vi "Get Controllers via Storage API.vi"(6 "Action":enum16{"PID", "Industrial"}(ring), 7 "VI reference (current VI)":refnum<vi>, 8 "error in (no error)":errorcluster, 10 "Tree":refnum<vi>, 11 "NIVS.System Definition Root":refnum<k24>) -> (0 "error out":errorcluster, 3 "NIVS.System Definition Root":refnum<k24>)   [LabVIEW 2019, in "Control Workspace Object.lvlib"]
uses:
  NationalInstruments.VeriStand.SystemStorage
  <vilib>/picture/picture.llb/imagedata.ctl
  Shared/Constants.vi
  Control Workspace Object.lvlib
  Workspace Shared/Control Workspace Shared.lvlib
  NationalInstruments.VeriStand.SystemDefinitionAPI
  Shared/Control Addon Shared.lvlib
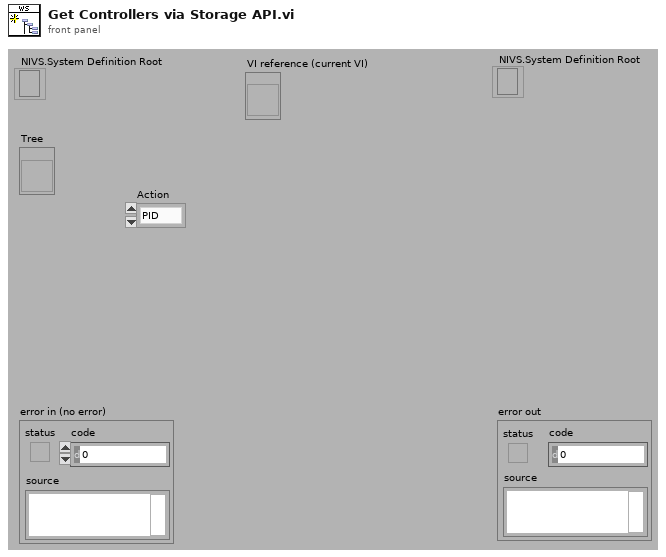
[diagram p1: front panel]
types:
  T1 = typedef "imagedata.ctl" = cluster{"image type":i32, "image depth":i32, "image":u8[], "mask":u8[], "colors":u32[], "Rectangle":cluster{"left":i16, "top":i16, "right":i16, "bottom":i16}}
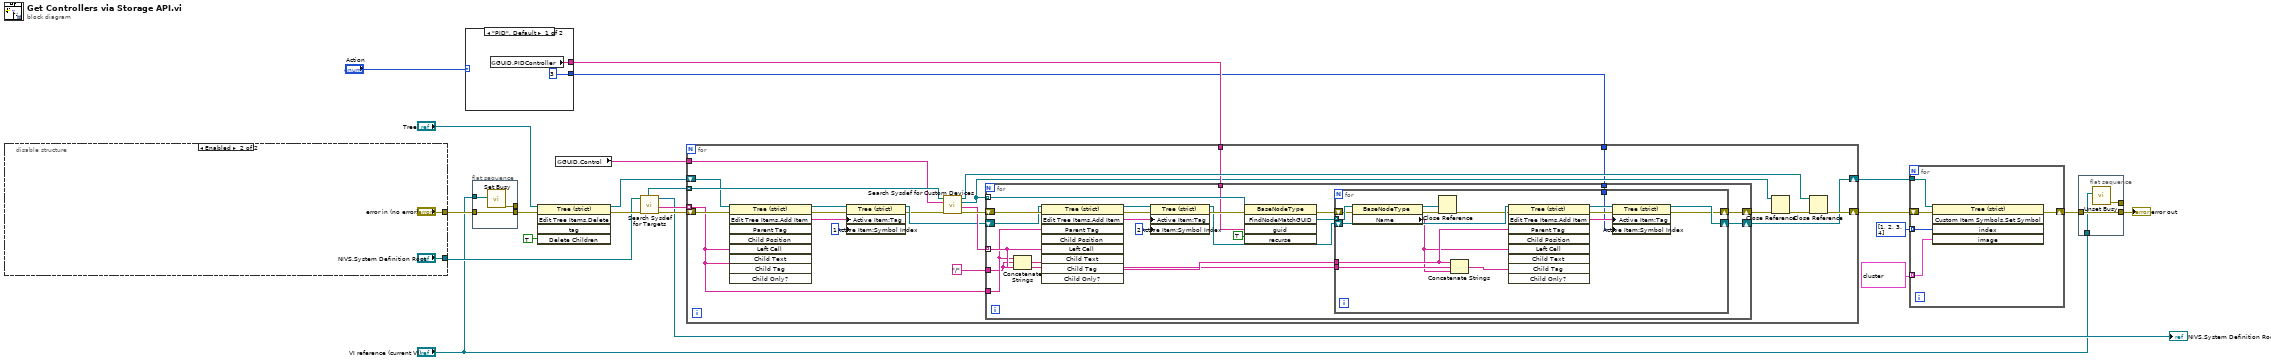
[diagram p0: block diagram]
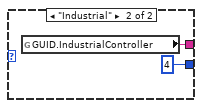
[diagram p2: hidden frame]
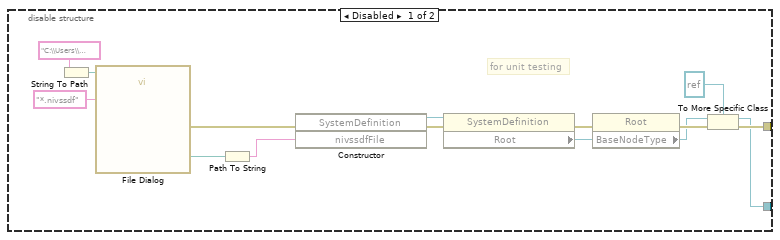
[diagram p3: hidden frame]
diagram:
  n1 = disable-structure shown="Enabled" {
    disable-tunnel: [w24 "NIVS.System Definition Root"] -> w14
    disable-tunnel: [w29 "error in (no error)"] -> w6
    frame Disabled {
      # "for unit testing"
      n2 = String To Path(string="C:\\Users\\Public\\Documents\\National Instruments\\NI VeriStand 2010\\Projects") -> (path=w25:path)
      n3 = call "File Dialog"("start path"=w25, "pattern (all files)"="*.nivssdf") -> ("selected path"=w36:path, "error out"=w23:errorcluster)  [unwired: 10 in, 2 out]
      n4 = Path To String(path=w36) -> (string=w35:string)
      n5 = constructor class="SystemDefinition"(error in=w23, "nivssdfFile"=w35) -> (reference out=w33:refnum<k24>, error out=w34:errorcluster)  [unwired: 2 in, 2 out]
      n6 = property class="SystemDefinition"(reference=w33, error in=w34) -> (error out=w31:errorcluster, "Root"=w32:refnum<k24>)  [unwired: 1 out]
      n7 = property class="Root"(reference=w32, error in=w31) -> (error out=w30:errorcluster, "BaseNodeType"=w28:refnum<k24>)  [unwired: 1 out]
      n8 = To More Specific Class(target class=refnum<k24> refnum, reference=w28, error in=w30) -> (specific class reference=w24:refnum<k24>, error out=w29:errorcluster)
    }
    frame Enabled {
    }
  }
  n9 = case shown="\"PID\", Default" "Action" {
    tunnel: [w41 w43] -> w4
    tunnel: [3 4] -> w2
    frame "PID", Default {
      n10 = global read "Constants.vi" "GUID.PIDController"() -> (w41:string)
    }
    frame "Industrial" {
      n11 = global read "Constants.vi" "GUID.IndustrialController"() -> (w43:string)
    }
  }
  n12 = flat-sequence {
    tunnel: [w45] -> w20
    tunnel: "VI reference (current VI)" -> [w46]
    tunnel: w6 -> [w45]
    tunnel: [w44] -> _
    frame #0 {
      n13 = call <vilib>:"Set Busy.vi"("VI reference (current VI)"=w46) -> ("error out"=w44:errorcluster)  [unwired: 9 in, 1 out]
    }
  }
  n14 = invoke class="Tree (strict)" method="Edit Tree Items.Delete"(reference="Tree", error in=w20, "Delete Children"=TRUE ("Delete Children?")) -> (reference out=w13:refnum<vi>, error out=w19:errorcluster)  [unwired: 2 in, 3 out]
  n15 = global read "Constants.vi" "GUID.Control"() -> (w1:string)
  n16 = call "Search Sysdef for Targets.vi"("error in (no error)"=w19, "NIVS.System Definition Root"=w14) -> ("error out"=w18:errorcluster, "Target Names"=w22:string[], "NIVS.System Defintion Root Out"=→"NIVS.System Definition Root":refnum<k24>, "Target Nodes"=w17:refnum<k24>[])  [unwired: 6 in]
  n17 = for {
    tunnel: w17 -> [w67] mode=indexing
    tunnel: w22 -> [w60] mode=indexing
    shift-right: [w62] -> w11
    shift-left: w18 -> [w68]
    tunnel: w1 -> [w58]
    shift-right: [w51] -> w12
    shift-left: w13 -> [w50]
    tunnel: w4 -> [w49]
    tunnel: w2 -> [w47]
    n18 = invoke class="Tree (strict)" method="Edit Tree Items.Add Item"(reference=w50, error in=w68, "Left Cell"=w60, "Child Tag"=w60) -> (reference out=w56:refnum<vi>, error out=w53:errorcluster, "Edit Tree Items:Add Item"=w54:string)  [unwired: 5 in, 6 out]
    n19 = property class="Tree (strict)"(reference=w56, error in=w53, "Active Item:Tag"=w54, "Active Item:Symbol Index"=1) -> (reference out=w55:refnum<vi>, error out=w52:errorcluster)
    n20 = call "Search Sysdef for Custom Devices.vi"("error in (no error)"=w52, "CD GUID"=w58, "Target Node"=w67) -> ("error out"=w66:errorcluster, "Custom Device Names"=w65:string[], "Custom Device Nodes"=w48:refnum<k24>[], "Target Node Out"=w61:refnum<k24>)  [unwired: 5 in]
    n21 = for {
      tunnel: w65 -> [w87] mode=indexing
      tunnel: w60 -> [w85]
      shift-right: [w73] -> w64
      shift-left: w66 -> [w88]
      tunnel: "/" ("string") -> [w70]
      shift-right: [w75] -> w51
      shift-left: w55 -> [w86]
      tunnel: w48 -> [w80] mode=indexing
      tunnel: w49 -> [w77]
      tunnel: w47 -> [w69]
      n22 = Concatenate Strings(w85, w70, w87) -> (w71:string)
      n23 = invoke class="Tree (strict)" method="Edit Tree Items.Add Item"(reference=w86, error in=w88, "Parent Tag"=w85, "Left Cell"=w87, "Child Tag"=w71) -> (reference out=w83:refnum<vi>, error out=w81:errorcluster, "Edit Tree Items:Add Item"=w82:string)  [unwired: 4 in, 6 out]
      n24 = property class="Tree (strict)"(reference=w83, error in=w81, "Active Item:Tag"=w82, "Active Item:Symbol Index"=2) -> (reference out=w76:refnum<vi>, error out=w79:errorcluster)
      n25 = invoke class="BaseNodeType" method="FindNodeMatchGUID"(reference=w80, error in=w79, "guid"=w77, "recurse"=TRUE) -> (error out=w74:errorcluster, "FindNodeMatchGUID"=w72:refnum<k24>[])  [unwired: 1 in, 3 out]
      n26 = for {
        shift-right: [w93] -> w75
        shift-left: w76 -> [w104]
        shift-right: [w91] -> w73
        shift-left: w74 -> [w102]
        tunnel: w72 -> [w103] mode=indexing
        tunnel: w71 -> [w100]
        tunnel: w70 -> [w99]
        tunnel: w69 -> [w89]
        n27 = property class="BaseNodeType"(reference=w103, error in=w102) -> (reference out=w95:refnum<k24>, error out=w101:errorcluster, "Name"=w98:string)
        n28 = Close Reference(reference=w95, error in (no error)=w101) -> (error out=w96:errorcluster)
        n29 = Concatenate Strings(w100, w99, w98) -> (w97:string)
        n30 = invoke class="Tree (strict)" method="Edit Tree Items.Add Item"(reference=w104, error in=w96, "Parent Tag"=w100, "Left Cell"=w98, "Child Tag"=w97) -> (reference out=w94:refnum<vi>, error out=w92:errorcluster, "Edit Tree Items:Add Item"=w90:string)  [unwired: 4 in, 6 out]
        n31 = property class="Tree (strict)"(reference=w94, error in=w92, "Active Item:Tag"=w90, "Active Item:Symbol Index"=w89) -> (reference out=w93:refnum<vi>, error out=w91:errorcluster)
      }
    }
    n32 = Close Reference(reference=w48, error in (no error)=w64) -> (error out=w63:errorcluster)
    n33 = Close Reference(reference=w61, error in (no error)=w63) -> (error out=w62:errorcluster)
  }
  n34 = for {
    tunnel: w12 -> [w109]
    shift-right: [w108] -> w9
    shift-left: w11 -> [w106]
    tunnel: i32[] [1, 2, 3, 4] -> [w107] mode=indexing
    tunnel: T1[] [{"image type"=0, "image depth"=32, "image"=array[1024 elements], "mask"=[0, 0, 0, 0, 0, 0, 63, 254, 127, 254, 255, 254, 255, 255, 255, 255, 255, 255, 255, 255, 255, 255, 255, 255, 127, 254, 64, 32, 0, 0, 0, 0], "colors"=[], "Rectangle"={"left"=0, "top"=0, "right"=16, "bottom"=16}}, {"image type"=0, "image depth"=32, "image"=array[1024 elements], "mask"=[255, 255, 255, 255, 255, 255, 255, 255, 255, 255, 255, 255, 255, 255, 255, 255, 255, 255, 255, 255, 255, 255, 255, 255, 255, 255, 255, 255, 255, 255, 255, 255], "colors"=[], "Rectangle"={"left"=0, "top"=0, "right"=16, "bottom"=16}}, {"image type"=0, "image depth"=32, "image"=[255, 255, 255, 255, 255, 255, 255, 255, 255, 255, 255, 255, 255, 255, 255, 255, 255, 255, 255, 255, 255, 255, 255, 255, 255, 0, 0, 0, 255, 0, 0, 0, 255, 0, 0, 0, 255, 0, 0, 0, 255, 255, 255, 255, 255, 255, 255, 255, 255, 255, 255, 255, 255, 255, 255, 255, 255, 255, 255, 255, 255, 255, 255, 255, 255, 255, 255, 255, 255, 255, 255, 255, 255, 247, 247, 247, 255, 255, 255, 255, 255, 0, 0, 0, 255, 0, 0, 0, 255, 0, 0, 0, 255, 0, 0, 0, 255, 0, 0, 0, 255, 0, 0, 0, 255, 0, 0, 0, 255, 0, 0, 0, 255, 255, 255, 255, 255, 248, 248, 248, 255, 255, 255, 255, 255, 255, 255, 255, 255, 255, 255, 255, 255, 255, 255, 255, 255, 255, 255, 255, 255, 0, 0, 0, 255, 0, 0, 0, 255, 0, 0, 0, 255, 0, 0, 0, 255, 0, 0, 0, 255, 0, 0, 0, 255, 0, 0, 0, 255, 0, 0, 0, 255, 0, 0, 0, 255, 0, 0, 0, 255, 255, 255, 255, 255, 249, 249, 249, 255, 254, 254, 254, 255, 255, 255, 255, 255, 255, 255, 255, 255, 0, 0, 0, 255, 0, 0, 0, 255, 0, 0, 0, 255, 0, 0, 0, 255, 0, 0, 0, 255, 0, 0, 0, 255, 0, 0, 0, 255, 0, 0, 0, 255, 0, 0, 0, 255, 0, 0, 0, 255, 0, 0, 0, 255, 0, 0, 0, 255, 255, 255, 255, 255, 255, 255, 255, 255, 255, 255, 255, 255, 0, 0, 0, 255, 0, 0, 0, 255, 0, 0, 0, 255, 0, 0, 0, 255, 0, 0, 0, 255, 0, 0, 0, 255, 0, 0, 0, 255, 0, 0, 0, 255, 0, 0, 0, 255, 0, 0, 0, 255, 0, 0, 0, 255, 0, 0, 0, 255, 0, 0, 0, 255, 0, 0, 0, 255, 255, 255, 255, 255, 255, 255, 255, 255, 0, 0, 0, 255, 0, 0, 0, 255, 255, 255, 255, 255, 255, 255, 255, 255, 255, 255, 255, 255, 255, 255, 255, 255, 255, 255, 255, 255, 255, 255, 255, 255, 255, 255, 255, 255, 255, 255, 255, 255, 255, 255, 255, 255, 255, 255, 255, 255, 0, 0, 0, 255, 0, 0, 0, 255, 255, 255, 255, 255, 0, 0, 0, 255, 0, 0, 0, 255, 0, 0, 0, 255, 255, 255, 255, 255, 0, 0, 0, 255, 0, 0, 0, 255, 0, 0, 0, 255, 0, 0, 0, 255, 0, 0, 0, 255, 0, 0, 0, 255, 0, 0, 0, 255, 0, 0, 0, 255, 242, 242, 242, 255, 0, 0, 0, 255, 0, 0, 0, 255, 0, 0, 0, 255, 0, 0, 0, 255, 0, 0, 0, 255, 0, 0, 0, 255, 255, 255, 255, 255, 0, 0, 0, 255, 0, 0, 0, 255, 0, 0, 0, 255, 0, 0, 0, 255, 0, 0, 0, 255, 0, 0, 0, 255, 0, 0, 0, 255, 0, 0, 0, 255, 255, 255, 255, 255, 0, 0, 0, 255, 0, 0, 0, 255, 0, 0, 0, 255, 0, 0, 0, 255, 0, 0, 0, 255, 0, 0, 0, 255, 255, 255, 255, 255, 0, 0, 0, 255, 0, 0, 0, 255, 0, 0, 0, 255, 0, 0, 0, 255, 0, 0, 0, 255, 0, 0, 0, 255, 255, 255, 255, 255, 0, 0, 0, 255, 255, 255, 255, 255, 0, 0, 0, 255, 0, 0, 0, 255, 0, 0, 0, 255, 0, 0, 0, 255, 0, 0, 0, 255, 0, 0, 0, 255, 255, 255, 255, 255, 0, 0, 0, 255, 0, 0, 0, 255, 0, 0, 0, 255, 0, 0, 0, 255, 0, 0, 0, 255, 255, 255, 255, 255, 255, 255, 255, 255, 0, 0, 0, 255, 255, 255, 255, 255, 0, 0, 0, 255, 0, 0, 0, 255, 0, 0, 0, 255, 255, 255, 255, 255, 0, 0, 0, 255, 0, 0, 0, 255, 255, 255, 255, 255, 255, 255, 255, 255, 255, 255, 255, 255, 0, 0, 0, 255, 0, 0, 0, 255, 255, 255, 255, 255, 255, 255, 255, 255, 255, 255, 255, 255, 255, 255, 255, 255, 255, 255, 255, 255, 0, 0, 0, 255, 0, 0, 0, 255, 255, 255, 255, 255, 255, 255, 255, 255, 0, 0, 0, 255, 0, 0, 0, 255, 0, 0, 0, 255, 0, 0, 0, 255, 0, 0, 0, 255, 0, 0, 0, 255, 0, 0, 0, 255, 0, 0, 0, 255, 255, 255, 255, 255, 255, 255, 255, 255, 0, 0, 0, 255, 0, 0, 0, 255, 0, 0, 0, 255, 0, 0, 0, 255, 255, 255, 255, 255, 255, 255, 255, 255, 255, 255, 255, 255, 0, 0, 0, 255, 0, 0, 0, 255, 0, 0, 0, 255, 0, 0, 0, 255, 0, 0, 0, 255, 0, 0, 0, 255, 0, 0, 0, 255, 0, 0, 0, 255, 255, 255, 255, 255, 0, 0, 0, 255, 0, 0, 0, 255, 0, 0, 0, 255, 255, 255, 255, 255, 254, 254, 254, 255, 255, 255, 255, 255, 255, 255, 255, 255, 255, 255, 255, 255, 0, 0, 0, 255, 0, 0, 0, 255, 0, 0, 0, 255, 0, 0, 0, 255, 0, 0, 0, 255, 0, 0, 0, 255, 0, 0, 0, 255, 0, 0, 0, 255, 0, 0, 0, 255, 0, 0, 0, 255, 255, 255, 255, 255, 255, 255, 255, 255, 255, 255, 255, 255, 255, 255, 255, 255, 255, 255, 255, 255, 249, 249, 249, 255, 255, 255, 255, 255, 0, 0, 0, 255, 0, 0, 0, 255, 0, 0, 0, 255, 0, 0, 0, 255, 0, 0, 0, 255, 0, 0, 0, 255, 0, 0, 0, 255, 0, 0, 0, 255, 255, 255, 255, 255, 255, 255, 255, 255, 248, 248, 248, 255, 251, 251, 251, 255, 255, 255, 255, 255, 255, 255, 255, 255, 255, 255, 255, 255, 252, 252, 252, 255, 255, 255, 255, 255, 255, 255, 255, 255, 0, 0, 0, 255, 0, 0, 0, 255, 0, 0, 0, 255, 0, 0, 0, 255, 255, 255, 255, 255, 255, 255, 255, 255, 254, 254, 254, 255, 252, 252, 252, 255, 251, 251, 251, 255, 252, 252, 252], "mask"=[255, 255, 255, 255, 255, 255, 255, 255, 255, 255, 255, 255, 255, 255, 255, 255, 255, 255, 255, 255, 255, 255, 255, 255, 255, 255, 255, 255, 255, 255, 255, 255], "colors"=[], "Rectangle"={"left"=0, "top"=0, "right"=16, "bottom"=16}}, {"image type"=0, "image depth"=32, "image"=[255, 255, 255, 255, 255, 255, 255, 255, 255, 255, 255, 255, 255, 255, 255, 255, 255, 255, 255, 255, 255, 255, 255, 255, 255, 0, 0, 0, 255, 0, 0, 0, 255, 0, 0, 0, 255, 0, 0, 0, 255, 255, 255, 255, 255, 255, 255, 255, 255, 255, 255, 255, 255, 255, 255, 255, 255, 255, 255, 255, 255, 255, 255, 255, 255, 255, 255, 255, 255, 255, 255, 255, 255, 255, 255, 255, 255, 255, 255, 255, 255, 0, 0, 0, 255, 0, 0, 0, 255, 0, 0, 0, 255, 8, 8, 8, 255, 0, 0, 0, 255, 1, 1, 1, 255, 0, 0, 0, 255, 1, 1, 1, 255, 255, 255, 255, 255, 247, 247, 247, 255, 255, 255, 255, 255, 255, 255, 255, 255, 255, 255, 255, 255, 255, 255, 255, 255, 255, 255, 255, 255, 0, 0, 0, 255, 0, 0, 0, 255, 0, 0, 0, 255, 9, 9, 9, 255, 255, 255, 255, 255, 255, 255, 255, 255, 0, 0, 0, 255, 0, 0, 0, 255, 0, 0, 0, 255, 0, 0, 0, 255, 255, 255, 255, 255, 248, 248, 248, 255, 254, 254, 254, 255, 255, 255, 255, 255, 255, 255, 255, 255, 0, 0, 0, 255, 0, 0, 0, 255, 0, 0, 0, 255, 255, 255, 255, 255, 11, 11, 10, 255, 255, 255, 255, 255, 255, 255, 255, 255, 7, 7, 7, 255, 255, 255, 255, 255, 0, 0, 0, 255, 0, 0, 0, 255, 0, 0, 0, 255, 255, 255, 255, 255, 255, 255, 255, 255, 255, 255, 255, 255, 0, 0, 0, 255, 0, 0, 0, 255, 0, 0, 0, 255, 255, 255, 255, 255, 255, 255, 255, 255, 7, 7, 7, 255, 255, 255, 255, 255, 255, 255, 255, 255, 0, 0, 0, 255, 255, 255, 255, 255, 254, 254, 254, 255, 0, 0, 0, 255, 4, 4, 3, 255, 0, 0, 0, 255, 255, 255, 255, 255, 255, 255, 255, 255, 0, 0, 0, 255, 0, 0, 0, 255, 243, 243, 243, 255, 255, 255, 255, 255, 0, 0, 0, 255, 7, 7, 7, 255, 255, 255, 255, 255, 255, 255, 255, 255, 0, 0, 0, 255, 0, 0, 0, 255, 255, 255, 255, 255, 255, 255, 255, 255, 0, 0, 0, 255, 0, 0, 0, 255, 255, 255, 255, 255, 0, 0, 0, 255, 0, 0, 0, 255, 0, 0, 0, 255, 255, 255, 255, 255, 0, 0, 0, 255, 0, 0, 0, 255, 0, 0, 0, 255, 0, 0, 0, 255, 0, 0, 0, 255, 0, 0, 0, 255, 0, 0, 0, 255, 0, 0, 0, 255, 255, 255, 255, 255, 0, 0, 0, 255, 0, 0, 0, 255, 0, 0, 0, 255, 0, 0, 0, 255, 0, 0, 0, 255, 0, 0, 0, 255, 255, 255, 255, 255, 0, 0, 0, 255, 0, 0, 0, 255, 0, 0, 0, 255, 0, 0, 0, 255, 0, 0, 0, 255, 4, 4, 3, 255, 4, 4, 4, 255, 0, 0, 0, 255, 255, 255, 255, 255, 0, 0, 0, 255, 0, 0, 0, 255, 0, 0, 0, 255, 0, 0, 0, 255, 0, 0, 0, 255, 0, 0, 0, 255, 255, 255, 255, 255, 0, 0, 0, 255, 0, 0, 0, 255, 0, 0, 0, 255, 0, 0, 0, 255, 0, 0, 0, 255, 0, 0, 0, 255, 0, 0, 0, 255, 0, 0, 0, 255, 255, 255, 255, 255, 0, 0, 0, 255, 0, 0, 0, 255, 0, 0, 0, 255, 0, 0, 0, 255, 0, 0, 0, 255, 0, 0, 0, 255, 255, 255, 255, 255, 0, 0, 0, 255, 0, 0, 0, 255, 0, 0, 0, 255, 0, 0, 0, 255, 0, 0, 0, 255, 0, 0, 0, 255, 0, 0, 0, 255, 0, 0, 0, 255, 255, 255, 255, 255, 0, 0, 0, 255, 0, 0, 0, 255, 0, 0, 0, 255, 255, 255, 255, 255, 0, 0, 0, 255, 0, 0, 0, 255, 255, 255, 255, 255, 255, 255, 255, 255, 0, 0, 0, 255, 0, 0, 0, 255, 0, 0, 0, 255, 0, 0, 0, 255, 4, 4, 4, 255, 0, 0, 0, 255, 255, 255, 255, 255, 255, 255, 255, 255, 0, 0, 0, 255, 0, 0, 0, 255, 255, 255, 255, 255, 255, 255, 255, 255, 1, 1, 1, 255, 0, 0, 0, 255, 0, 0, 0, 255, 255, 255, 255, 255, 255, 255, 255, 255, 0, 0, 0, 255, 0, 0, 0, 255, 0, 0, 0, 255, 0, 0, 0, 255, 255, 255, 255, 255, 255, 255, 255, 255, 16, 16, 16, 255, 0, 0, 0, 255, 4, 4, 4, 255, 255, 255, 255, 255, 255, 255, 255, 255, 255, 255, 255, 255, 0, 0, 0, 255, 0, 0, 0, 255, 0, 0, 0, 255, 255, 255, 255, 255, 255, 255, 255, 255, 255, 255, 255, 255, 255, 255, 255, 255, 248, 248, 248, 255, 255, 255, 255, 255, 16, 16, 16, 255, 0, 0, 0, 255, 0, 0, 0, 255, 255, 255, 255, 255, 255, 255, 255, 255, 255, 255, 255, 255, 247, 247, 247, 255, 255, 255, 255, 255, 0, 0, 0, 255, 0, 0, 0, 255, 0, 0, 0, 255, 0, 0, 0, 255, 0, 0, 0, 255, 0, 0, 0, 255, 0, 0, 0, 255, 0, 0, 0, 255, 0, 0, 0, 255, 0, 0, 0, 255, 255, 255, 255, 255, 250, 250, 250, 255, 252, 252, 252, 255, 255, 255, 255, 255, 255, 255, 255, 255, 255, 255, 255, 255, 255, 255, 255, 255, 4, 4, 4, 255, 3, 3, 3, 255, 0, 0, 0, 255, 0, 0, 0, 255, 0, 0, 0, 255, 0, 0, 0, 255, 0, 0, 0, 255, 0, 0, 0, 255, 255, 255, 255, 255, 250, 250, 250, 255, 248, 248, 248, 255, 251, 251, 251, 255, 255, 255, 255, 255, 255, 255, 255, 255, 255, 255, 255, 255, 255, 255, 255, 255, 255, 255, 255, 255, 255, 255, 255, 255, 0, 0, 0, 255, 0, 0, 0, 255, 0, 0, 0, 255, 0, 0, 0, 255, 255, 255, 255, 255, 255, 255, 255, 255, 255, 255, 255, 255, 255, 255, 255, 255, 255, 255, 255, 255, 255, 255, 255], "mask"=[255, 255, 255, 255, 255, 255, 255, 255, 255, 255, 255, 255, 255, 255, 255, 255, 255, 255, 255, 255, 255, 255, 255, 255, 255, 255, 255, 255, 255, 255, 255, 255], "colors"=[], "Rectangle"={"left"=0, "top"=0, "right"=16, "bottom"=16}}] ("Array") -> [w105] mode=indexing
    n35 = invoke on="Invoke Node" class="Tree (strict)" method="Custom Item Symbols.Set Symbol"(reference=w109, error in=w106, "index"=w107, "image"=w105) -> (error out=w108:errorcluster)  [unwired: 1 in, 4 out]
  }
  n36 = flat-sequence {
    tunnel: w9 -> [w112]
    tunnel: [w112] -> w15
    tunnel: [w111] -> _
    tunnel: "VI reference (current VI)" -> [w110]
    frame #0 {
      n37 = call <vilib>:"Unset Busy.vi"("VI reference (current VI)"=w110) -> ("error out"=w111:errorcluster)  [unwired: 10 in]
    }
  }
  "error out" <- w15
